vi "carwash_test.vi"() -> ()   [LabVIEW 2017]
panel:
  out "?":bool
  out "?":bool
  out "?":bool
  out "Vehicle Out of Position":bool
  out "Air Dry":bool
  out "Clear Water Rinse":bool
  out "Main High Press. Wash":bool
  out "Soap Application":bool
  out "Under body Wash":bool
  in  "?":bool
  in  "?":bool
  in  "?":bool
  in  "stop":bool
  # "Car Wash Indicators"
  # "Underbody wash\nposition \nSwitch"
  # "Main Wash \nPosition \nSwitch"
  # "Air Dry\nPosition\nSwitch"
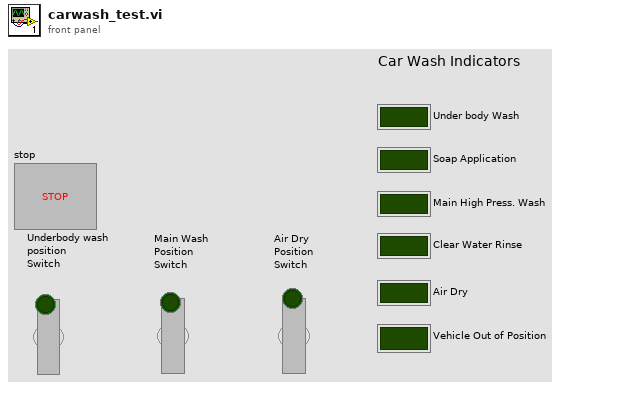
[diagram p1: front panel]
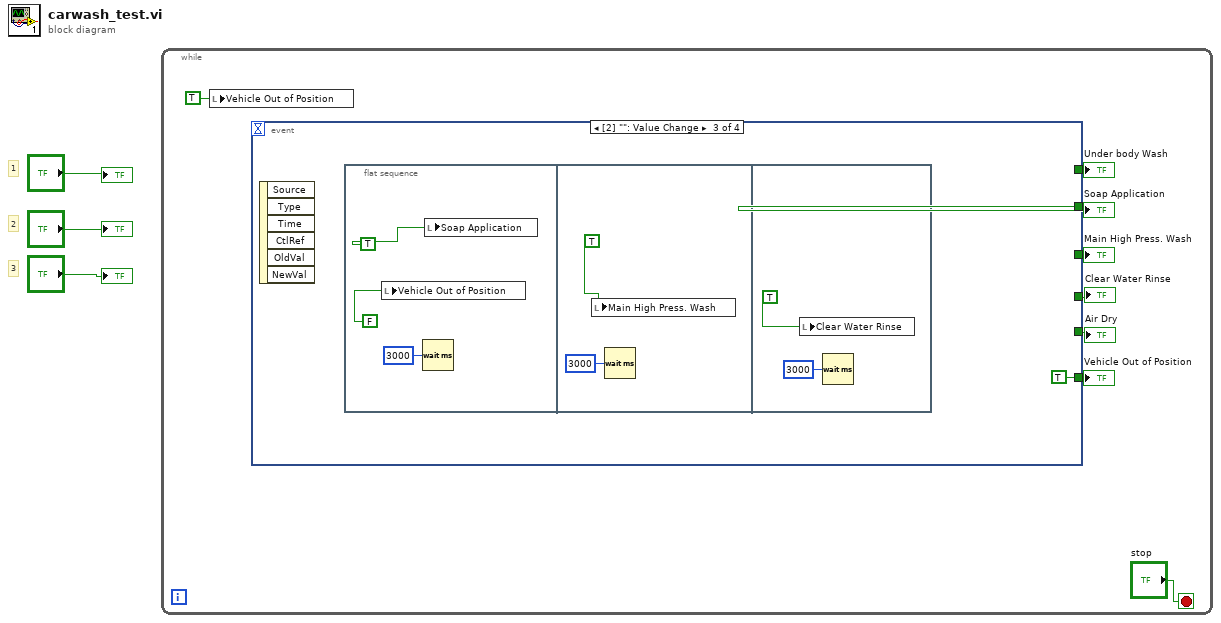
[diagram p0: block diagram]
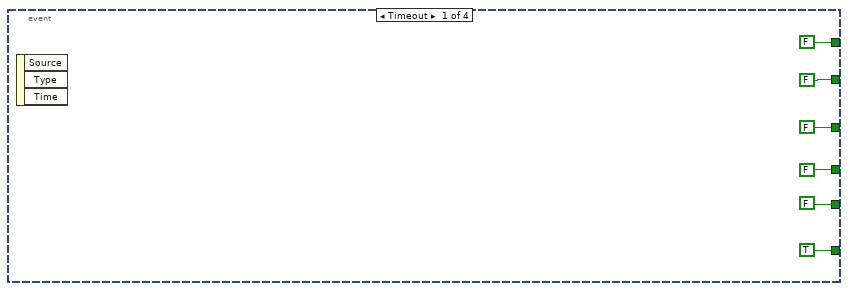
[diagram p2: hidden frame]
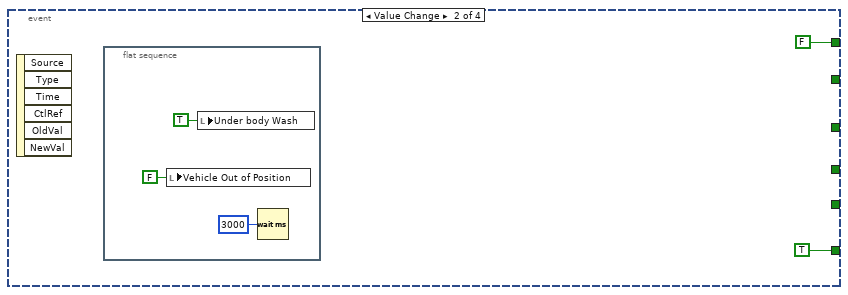
[diagram p3: hidden frame]
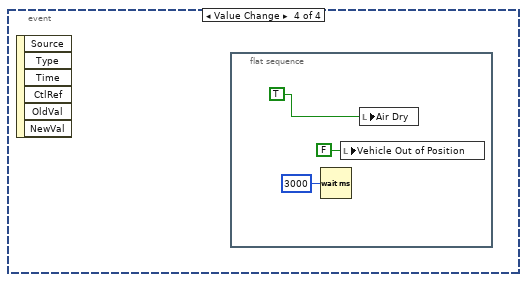
[diagram p4: hidden frame]
diagram:
  # "3"
  # "1"
  # "2"
  n1 = while {
    stop <- "stop" stop-if-true
    n2 = local write "Vehicle Out of Position"(TRUE ("Vehicle Out of Position")) -> ()
    n3 = event shown="[2] \"\": Value Change" {
      selector: _ -> [_ _ _ _]
      dyn-events: _ -> [_ _ _ _]
      timeout: _ -> [_ _ _ _]
      tunnel: [FALSE FALSE _ _] -> w10
      tunnel: [FALSE _ _ _] -> w9
      tunnel: [FALSE _ _ _] -> w8
      tunnel: [FALSE _ _ _] -> w7
      tunnel: [FALSE _ _ _] -> w6
      tunnel: [TRUE TRUE TRUE _] -> w5
      event Timeout {
        n4 = event-data() -> ()  [unwired: 1 in, 3 out]
      }
      event Value Change {
        n5 = event-data() -> ()  [unwired: 1 in, 6 out]
        n6 = flat-sequence {
          frame #0 {
            n7 = local write "Vehicle Out of Position"(FALSE ("Vehicle Out of Position")) -> ()
            n8 = local write "Under body Wash"(TRUE ("Under body Wash")) -> ()
            n9 = Wait (ms)(milliseconds to wait=u32 3000) -> ()  [unwired: 1 out]
          }
        }
      }
      event Value Change {
        n10 = event-data() -> ()  [unwired: 1 in, 6 out]
        n11 = flat-sequence {
          frame #0 {
            n12 = local write "Vehicle Out of Position"(FALSE ("Vehicle Out of Position")) -> ()
            n13 = Wait (ms)(milliseconds to wait=u32 3000) -> ()  [unwired: 1 out]
            n14 = local write "Soap Application"(TRUE ("Boolean 2")) -> ()
          }
          frame #1 {
            n15 = local write "Main High Press. Wash"(TRUE ("Boolean 4")) -> ()
            n16 = Wait (ms)(milliseconds to wait=u32 3000) -> ()  [unwired: 1 out]
          }
          frame #2 {
            n17 = local write "Clear Water Rinse"(TRUE ("Boolean 4")) -> ()
            n18 = Wait (ms)(milliseconds to wait=u32 3000) -> ()  [unwired: 1 out]
          }
        }
      }
      event Value Change {
        n19 = event-data() -> ()  [unwired: 1 in, 6 out]
        n20 = flat-sequence {
          frame #0 {
            n21 = Wait (ms)(milliseconds to wait=u32 3000) -> ()  [unwired: 1 out]
            n22 = local write "Vehicle Out of Position"(FALSE ("Vehicle Out of Position")) -> ()
            n23 = local write "Air Dry"(TRUE ("Air Dry")) -> ()
          }
        }
      }
    }
    "Under body Wash" <- w10
    "Soap Application" <- w9
    "Main High Press. Wash" <- w8
    "Clear Water Rinse" <- w7
    "Air Dry" <- w6
    "Vehicle Out of Position" <- w5
  }
  "?" <- "?"
  "?" <- "?"
  "?" <- "?"
